vi "CFTS-Init State.vi"(0 "Experimenter":string, 5 "Num":i32, 7 "Right":string, 9 "Left":string) -> (4 "State (out)":T1, 15 "error out":errorcluster)   [LabVIEW 2020]
doc: "Initializes ABI experiment state based on the specified experiment ID."
uses:
  CFTS-Experiment State.ctl
  CFTS-Globals.vi
panel:
  in  "Root folder":path
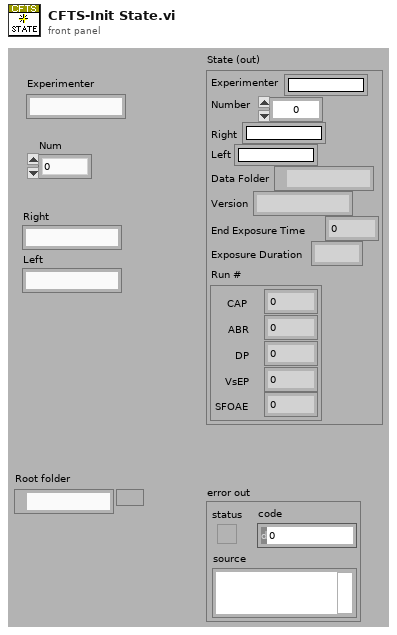
[diagram p1: front panel]
types:
  T1 = typedef "CFTS-Experiment State.ctl" = cluster{"Experimenter":string, "Number":u32, "Right":string, "Left":string, "Data Folder":path, "Version":string, "End Exposure Time":dbl, "Exposure Duration":string, "Run #":cluster{"CAP":i32, "ABR":i32, "DP":i32, "VsEP":i32, "SFOAE":i32}}
  T2 = cluster{"CAP":i16, "ABR":i16, "DP":i16, "VsEP":i16, "MeasSeq 3":i16}
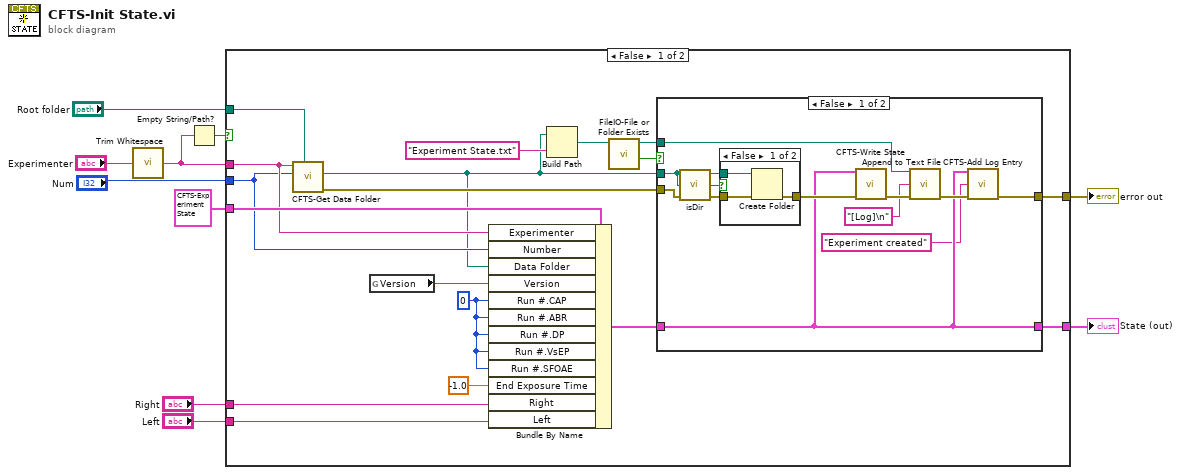
[diagram p0: block diagram]
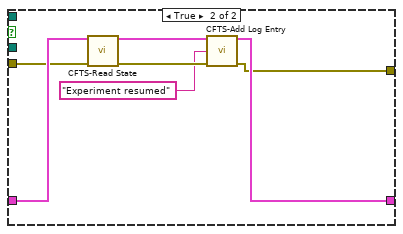
[diagram p3: hidden frame]
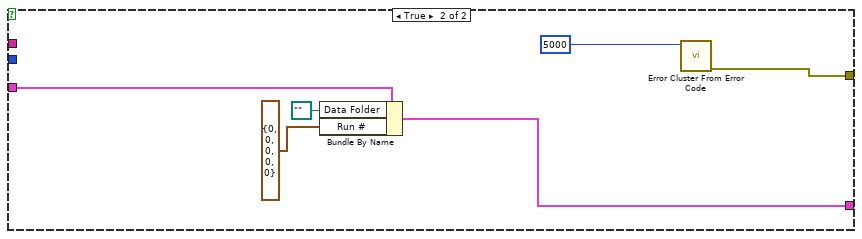
[diagram p4: hidden frame]
diagram:
  n1 = call <vilib>:"Trim Whitespace.vi"("string"="Experimenter") -> ("trimmed string"=w8:string)  [unwired: 1 in]
  n2 = Empty String/Path?(string/path=w8) -> (empty?=w9:bool)
  n3 = case shown="False" w9 {
    tunnel: T1 {"Experimenter"="", "Number"=0, "Right"="", "Left"="", "Data Folder"=path "", "Version"="", "End Exposure Time"=0.0, "Exposure Duration"="", "Run #"={"CAP"=0, "ABR"=0, "DP"=0, "VsEP"=0, "SFOAE"=0}} ("State") -> [w28 w56]
    tunnel: [w24 w53] -> w7
    tunnel: w8 -> [w25 _]
    tunnel: "Num" -> [w16 _]
    tunnel: [w23 w55] -> w10
    tunnel: "Root folder" -> [w20 _]
    tunnel: "Left" -> [w18 _]
    tunnel: "Right" -> [w17 _]
    frame False {
      w21 = 0 ("Next run #")
      n4 = call "CFTS-Get Data Folder.vi"("Root folder"=w20, "Number"=w16, "Experimenter"=w25) -> ("error out"=w22:errorcluster, "Data folder"=w14:path)  [unwired: 7 in]
      n5 = global read "CFTS-Globals.vi" "Version"() -> (w19:string)
      n6 = Bundle By Name(cluster=w28, "Experimenter"=w25, "Number"=w16, "Data Folder"=w14, "Version"=w19, "Run #.CAP"=w21, "Run #.ABR"=w21, "Run #.DP"=w21, "Run #.VsEP"=w21, "Run #.SFOAE"=w21, "End Exposure Time"=-1.0, "Right"=w17, "Left"=w18) -> (w27:T1)
      n7 = Build Path(base path=w14, name or relative path="Experiment State.txt" ("subkey")) -> (appended path=w13:path)
      n8 = call "FileIO-File or Folder Exists.vi"("path"=w13) -> ("Exists?"=w12:bool, "dup path"=w11:path)  [unwired: 7 in, 2 out]
      n9 = case shown="False" w12 {
        tunnel: w14 -> [w36 _]
        tunnel: [w31 w45] -> w24
        tunnel: w27 -> [w30 w50]
        tunnel: [w30 w46] -> w23
        tunnel: w22 -> [w38 w49]
        tunnel: w11 -> [w34 _]
        frame False {
          n10 = call "isDir.vi"("path"=w36) -> ("is Dir?"=w35:bool)
          n11 = case shown="False" w35 {
            tunnel: [w42 w43] -> w39
            tunnel: w38 -> [w41 w43]
            tunnel: w36 -> [w40 _]
            frame False {
              n12 = Create Folder(path (use dialog)=w40, error in=w41) -> (error out=w42:errorcluster)  [unwired: 1 in, 2 out]
            }
            frame True {
            }
          }
          n13 = call "CFTS-Write State.vi"("State"=w30, "error in (no error)"=w39) -> ("error out"=w37:errorcluster)  [unwired: 13 in]
          n14 = call "Append to Text File.vi"("file path"=w34, "text"="[Log]\n", "error in (no error)"=w37) -> ("error out"=w32:errorcluster)  [unwired: 11 in, 1 out]
          n15 = call "CFTS-Add Log Entry.vi"("State"=w30, "message"="Experiment created", "error in (no error)"=w32) -> ("error out"=w31:errorcluster)  [unwired: 11 in, 1 out]
        }
        frame True {
          n16 = call "CFTS-Read State.vi"("State In"=w50, "error in (no error)"=w49) -> ("State Out"=w47:T1, "error out"=w48:errorcluster)  [unwired: 12 in]
          n17 = call "CFTS-Add Log Entry.vi"("State"=w47, "message"="Experiment resumed", "error in (no error)"=w48) -> ("State thru"=w46:T1, "error out"=w45:errorcluster)  [unwired: 11 in]
        }
      }
    }
    frame True {
      n18 = Bundle By Name(cluster=w56, "Data Folder"=path "", "Run #"=T2 {"CAP"=0, "ABR"=0, "DP"=0, "VsEP"=0, "MeasSeq 3"=0}) -> (w55:T1)
      n19 = call <vilib>:"Error Cluster From Error Code.vi"("error code (0)"=5000) -> ("error out"=w53:errorcluster)  [unwired: 8 in]
    }
  }
  "State (out)" <- w10
  "error out" <- w7
